vi "Get VIAnalyzerConfiguration.vi"(8 "error in":errorcluster, 11 "DOM document in":refnum<k20>) -> (0 "error out":errorcluster, 2 "Element":refnum<k20>, 3 "DOM document out":refnum<k20>)   [LabVIEW 2020]
uses:
  <resource>/objmgr/DOMUserDefRef.rc
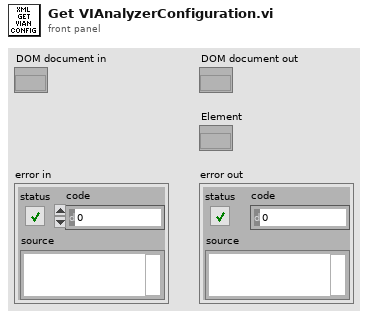
[diagram p1: front panel]
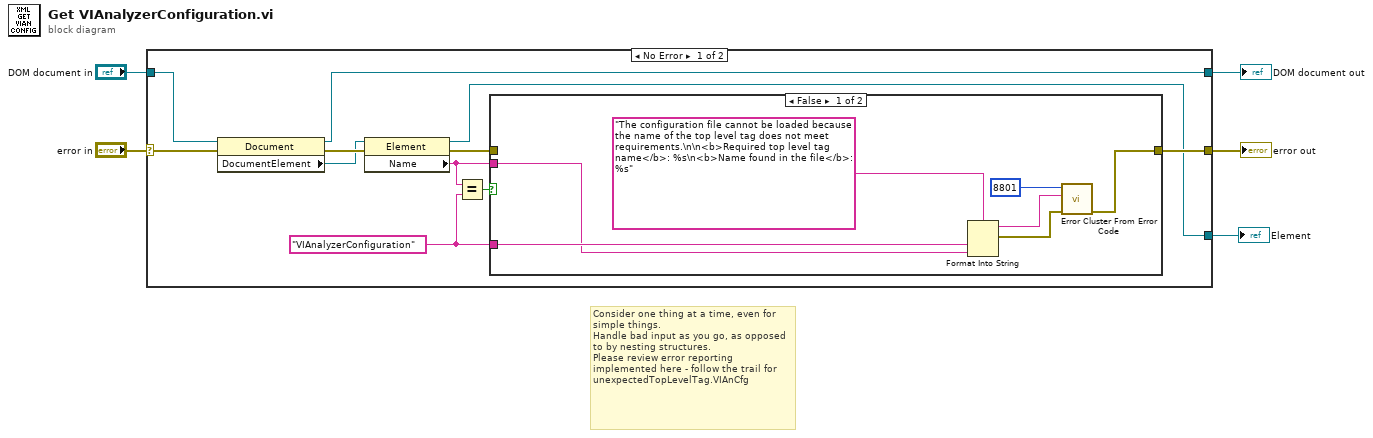
[diagram p0: block diagram]
diagram:
  # "Consider one thing at a time, even for simple things.\nHandle bad input as you go, as opposed to by nesting structures.\nPlease review error reporting implemented here - follow the trail for unexpectedTopLevelTag.VIAnCfg"
  n1 = case shown="No Error" "error in" {
    selector: "error in" -> [w14 w26]
    tunnel: [w6 w25] -> w5
    tunnel: [w16 w26] -> w4
    tunnel: "DOM document in" -> [w15 w25]
    tunnel: [w9 _] -> w1
    frame No Error {
      w8 = "VIAnalyzerConfiguration" ("Tag Name")
      n2 = property class="Document"(reference=w15, error in=w14) -> (reference out=w6:refnum<k20>, error out=w13:errorcluster, "DocumentElement"=w12:refnum<k20>)
      n3 = property class="Element"(reference=w12, error in=w13) -> (reference out=w9:refnum<k20>, error out=w10:errorcluster, "Name"=w7:string)
      n4 = Equal?(x=w7, y=w8) -> (x = y?=w11:bool)
      n5 = case shown="False" w11 {
        tunnel: [w17 w24] -> w16
        tunnel: w10 -> [_ w24]
        tunnel: w8 -> [w22 _]
        tunnel: w7 -> [w21 _]
        frame False {
          n6 = Format Into String(format string="The configuration file cannot be loaded because the name of the top level tag does not meet requirements.\n\n<b>Required top level tag name</b>: %s\n<b>Name found in the file</b>: %s", w22, w21) -> (resulting string=w19:string, error out=w18:errorcluster)  [unwired: 2 in]
          n7 = call <vilib>:"Error Cluster From Error Code.vi"("error in (no error)"=w18, "error message (\"\")"=w19, "error code (0)"=8801) -> ("error out"=w17:errorcluster)  [unwired: 6 in]
        }
        frame True {
        }
      }
    }
    frame Error {
    }
  }
  "DOM document out" <- w5
  "error out" <- w4
  "Element" <- w1
